vi "InitScope5761.vi"(6 "FpgaRef5782":refnum<class "FpgaRef5782.lvclass">, 8 "error in (no error)":errorcluster, 9 "FpgaRef5761 - 2":refnum<class "FpgaRef5761.lvclass">, 10 "FpgaRef5761 - 1":refnum<class "FpgaRef5761.lvclass">, 11 "Scope5761 in":refnum<class "Scope5761.lvclass">) -> (0 "error out":errorcluster, 3 "Scope5761 out":refnum<class "Scope5761.lvclass">)   [LabVIEW 2013, in "Scope5761.lvclass"]
uses:
  Scope5761.lvclass
  FpgaRef/FpgaRef5761/FpgaRef5761.lvclass
  FpgaRef/FpgaRef5782/FpgaRef5782.lvclass
  Scope5761.lvclass/Scope5761.ctl
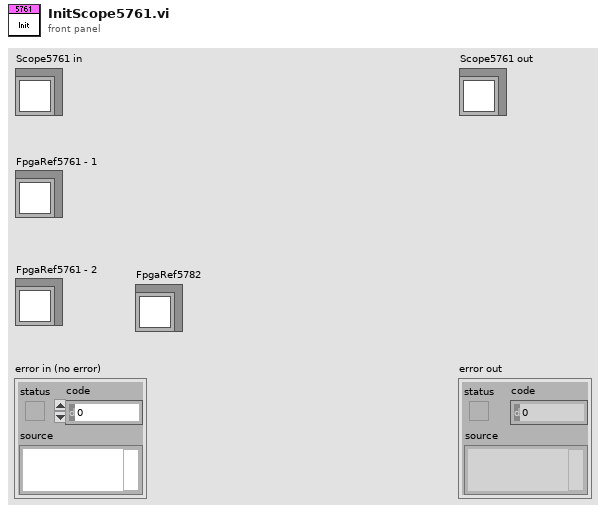
[diagram p1: front panel]
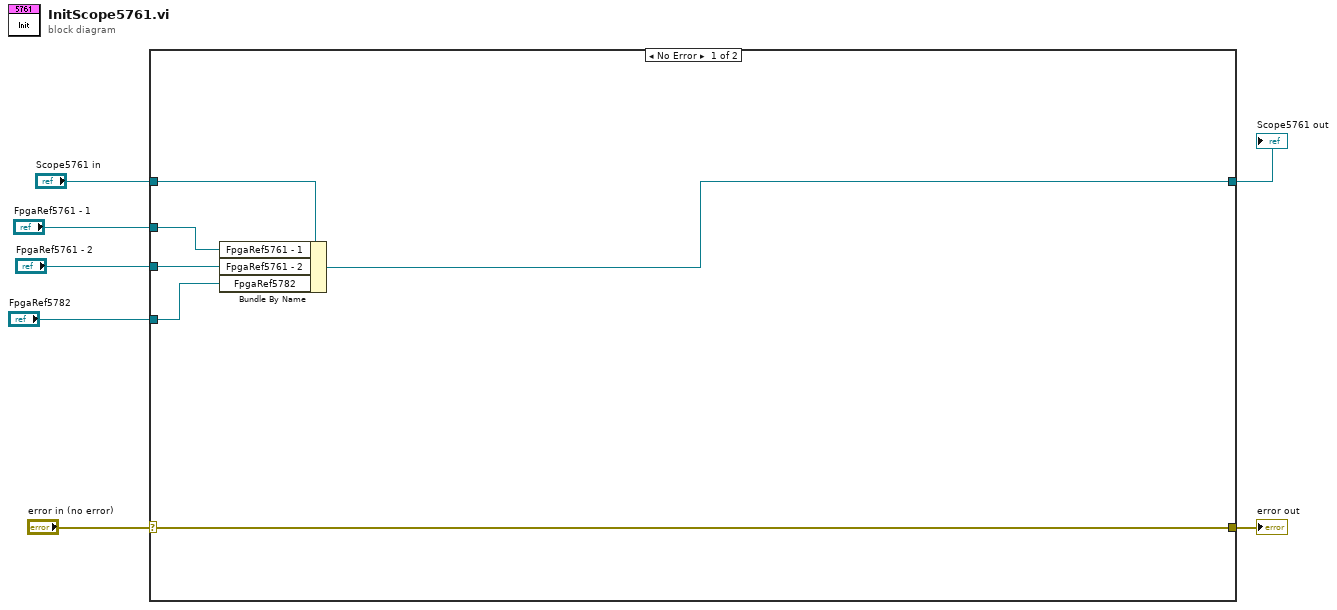
[diagram p0: block diagram]
diagram:
  n1 = case shown="No Error" "error in (no error)" {
    selector: "error in (no error)" -> [w13 w15]
    tunnel: [w13 w15] -> w6
    tunnel: "Scope5761 in" -> [w12 w14]
    tunnel: "FpgaRef5761 - 2" -> [w11 _]
    tunnel: "FpgaRef5761 - 1" -> [w10 _]
    tunnel: [w9 w14] -> w2
    tunnel: "FpgaRef5782" -> [w8 _]
    frame No Error {
      n2 = Bundle By Name(cluster=w12, "FpgaRef5761 - 1"=w10, "FpgaRef5761 - 2"=w11, "FpgaRef5782"=w8) -> (w9:refnum<class "Scope5761.lvclass">)
    }
    frame Error {
    }
  }
  "error out" <- w6
  "Scope5761 out" <- w2
